vi "Create Array of Tx Message Info.vi"(7 "error in":errorcluster, 8 "1553 channel handles":T7[](array[typedef]) {"terminal status channels" format="%.0x"; "error count channel refs"."wrong sync" format="%.0x"; "error count channel refs"."word" format="%.0x"; "error count channel refs"."unconfigured frames" format="%.0x"; "error count channel refs"."parity" format="%.0x"; "error count channel refs"."monitor" format="%.0x"; "error count channel refs"."Manchester" format="%.0x"; "error count channel refs"."improper number of words" format="%.0x"; "error count channel refs"."general protocol" format="%.0x"; "messages"."Rx status handles" format="%.0x"; "messages"."Tx status handles" format="%.0x"; "messages"."timestamps" format="%.0x"; "messages"."parameters"."RxBC channel handle" format="%.0x"; "messages"."parameters"."RxRT channel handle" format="%.0x"; "messages"."parameters"."Tx channel handle" format="%.0x"}, 9 "hardware handles":T12, 10 "1553 channels":T13[](array[typedef])) -> (0 "error out":errorcluster, 2 "transmitted messages":T1[](array[typedef]), 3 "array of message info":T6[](array[typedef]))   [LabVIEW 2023, in "Ballard MIL-STD-1553 Engine Support.lvlib" / "Custom Device.lvlib"]
uses:
  Custom Device.lvlib
  Shared/1553 Channel.ctl
  Shared/Address.ctl
  Shared/Message Definition.ctl
  Shared/Message Type.ctl
  Shared/Terminal Endpoint.ctl
  Shared/Parameter Definition.ctl
  Hardware Handles.ctl
  Implementation/Execution Unit/1553 Channel Handles.ctl
  Implementation/Execution Unit/Message Handles.ctl
  Implementation/Execution Unit/Parameter Handles.ctl
  <vilib>/NI VeriStand/Custom Device API/Custom Device Item Ref.ctl
  Shared/Error Count Channel Refs.ctl
  Shared/Tx Write Info.ctl
  <vilib>/NI VeriStand/Custom Device API/Custom Device API.lvlib
  Implementation/Execution Unit/Execution Unit.lvclass
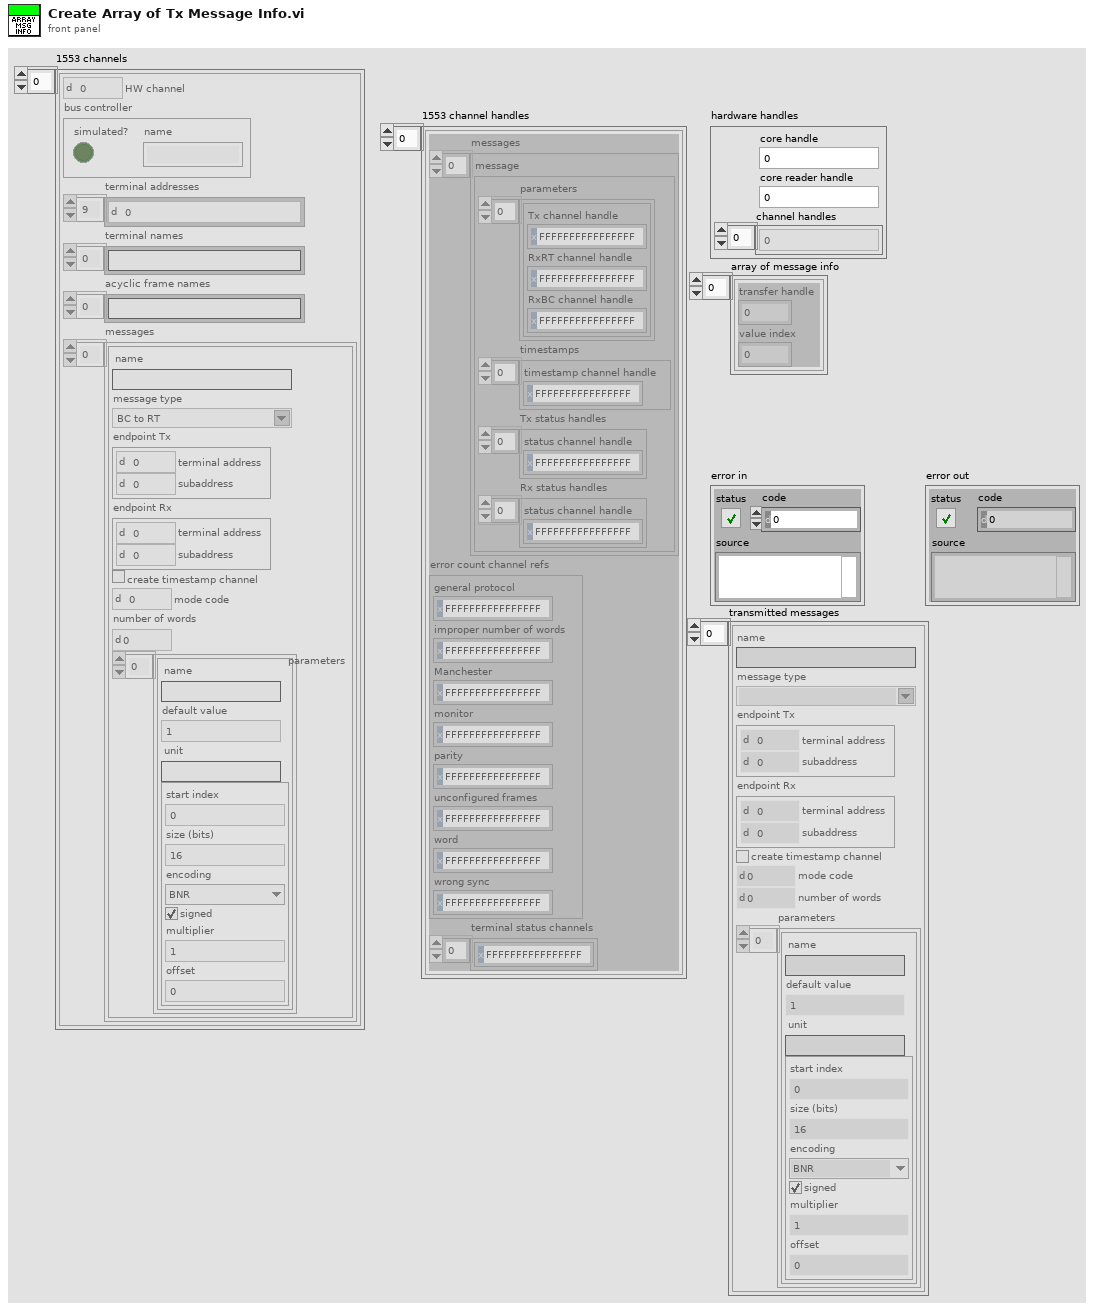
[diagram p1: front panel]
types:
  T1 = typedef "Message Definition.ctl" = cluster{"name":string, "message type":T2, "endpoint Tx":T3, "endpoint Rx":T3, "create timestamp channel":bool, "mode code":u16, "number of words":u16, "parameters":cluster{"name":string, "default value":dbl, "unit":string, "parameter definition":T5}[]}
  T2 = typedef "Message Type.ctl" = string
  T3 = typedef "Terminal Endpoint.ctl" = cluster{"terminal address":T4, "subaddress":T4}
  T4 = typedef "Address.ctl" = u16
  T5 = typedef "Parameter Definition.ctl" = cluster{"start index":i32, "size (bits)":i32, "encoding":enum16{"BNR", "BCD", "Discrete"}, "signed":bool, "multiplier":dbl, "offset":dbl}
  T6 = typedef "Tx Write Info.ctl" = cluster{"transfer handle":u64, "value index":i32}
  T7 = typedef "Ballard MIL-STD-1553 Engine Support.lvlib/Implementation.lvlib/Execution Unit.lvclass/1553 Channel Handles.ctl" = cluster{"messages":T8[], "error count channel refs":T11, "terminal status channels":T10[]}
  T8 = typedef "Ballard MIL-STD-1553 Engine Support.lvlib/Implementation.lvlib/Execution Unit.lvclass/Message Handles.ctl" = cluster{"parameters":T9[], "timestamps":T10[], "Tx status handles":T10[], "Rx status handles":T10[]}
  T9 = typedef "Ballard MIL-STD-1553 Engine Support.lvlib/Implementation.lvlib/Execution Unit.lvclass/Parameter Handles.ctl" = cluster{"Tx channel handle":T10, "RxRT channel handle":T10, "RxBC channel handle":T10}
  T10 = typedef "Custom Device API.lvlib/Custom Device Item Ref.ctl" = u64
  T11 = typedef "Error Count Channel Refs.ctl" = cluster{"general protocol":T10, "improper number of words":T10, "Manchester":T10, "monitor":T10, "parity":T10, "unconfigured frames":T10, "word":T10, "wrong sync":T10}
  T12 = typedef "Ballard MIL-STD-1553 Engine Support.lvlib/Custom Device.lvlib/Hardware Handles.ctl" = cluster{"core handle":u64, "core reader handle":u64, "channel handles":u64[]}
  T13 = typedef "1553 Channel.ctl" = cluster{"HW channel":u16, "bus controller":cluster{"simulated?":bool, "name":string}, "terminal addresses":T4[], "terminal names":string[], "acyclic frame names":string[], "messages":T1[]}
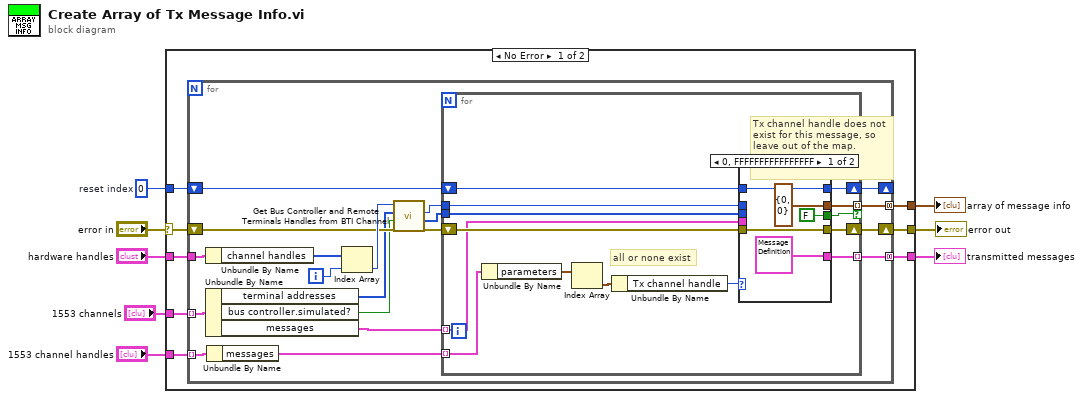
[diagram p0: block diagram]
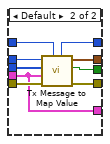
[diagram p2: hidden frame]
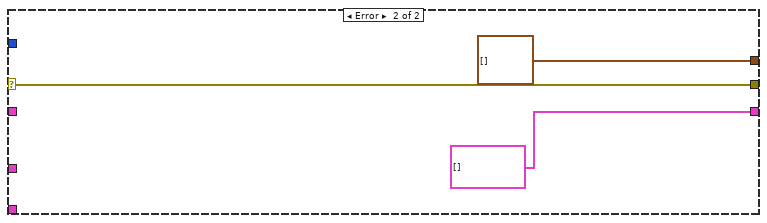
[diagram p3: hidden frame]
diagram:
  w3 = 0  # reset index
  n1 = case shown="No Error" "error in" {
    selector: "error in" -> [w15 w66]
    tunnel: "1553 channels" -> [w12 _]
    tunnel: "hardware handles" -> [w16 _]
    tunnel: [w14 w66] -> w5
    tunnel: "1553 channel handles" -> [w13 _]
    tunnel: w3 -> [w11 _]
    tunnel: [w10 T1[] []] -> w2
    tunnel: [w9 T6[] []] -> w1
    frame No Error {
      n2 = for {
        tunnel: w12 -> [w35] mode=indexing
        tunnel: w16 -> [w33]
        shift-right: [w31] -> w14
        shift-left: w15 -> [w27]
        tunnel: w13 -> [w30] mode=indexing
        shift-right: [w25] -> _
        shift-left: w11 -> [w26]
        tunnel: [w19] -> w10 mode=concatenating
        tunnel: [w18] -> w9 mode=concatenating
        i -> [w20]
        n3 = Unbundle By Name(w33) -> ("channel handles"=w21:u64[])
        n4 = Unbundle By Name(w35) -> ("terminal addresses"=w22:T4[], "bus controller.simulated?"=w17:bool, "messages"=w34:T1[])
        n5 = Unbundle By Name(w30) -> ("messages"=w29:T8[])
        n6 = Index Array(array=w21, index=w20) -> (element=w28:u64)
        n7 = call "Get Bus Controller and Remote Terminals Handles from BTI Channel.vi"("error in"=w27, "bus controller?"=w17, "terminal addresses"=w22, "channel handle in"=w28) -> ("error out"=w32:errorcluster, "remote terminal handles out"=w23:u64[], "bus controller handle out"=w24:u64)  [unwired: 4 in, 1 out]
        n8 = for {
          tunnel: w34 -> [w39] mode=indexing
          shift-right: [w49] -> w31
          shift-left: w32 -> [w42]
          tunnel: w23 -> [w48]
          tunnel: w29 -> [w47] mode=indexing
          tunnel: w24 -> [w43]
          shift-right: [w40] -> w25
          shift-left: w26 -> [w41]
          tunnel: [w37] -> w19 mode=indexing
          tunnel: [w38] -> w18 mode=indexing if=w36
          # "all or none exist"
          n9 = Unbundle By Name(w47) -> ("parameters"=w46:T9[])
          n10 = Index Array(array=w46) -> (element=w45:T9)  [unwired: 1 in]
          n11 = Unbundle By Name(w45) -> ("Tx channel handle"=w44:T10)
          n12 = case shown="0, FFFFFFFFFFFFFFFF" w44 {
            tunnel: w42 -> [w54 w63]
            tunnel: [w54 w62] -> w49
            tunnel: w48 -> [_ w61]
            tunnel: w39 -> [_ w56]
            tunnel: w43 -> [_ w60]
            tunnel: w41 -> [w53 w59]
            tunnel: [w53 w58] -> w40
            tunnel: [T6 {"transfer handle"=0, "value index"=0} ("Tx write info") w57] -> w38
            tunnel: [T1 {"name"="", "message type"="BC to RT", "endpoint Tx"={"terminal address"=0, "subaddress"=0}, "endpoint Rx"={"terminal address"=0, "subaddress"=0}, "create timestamp channel"=FALSE, "mode code"=0, "number of words"=0, "parameters"=[]} w56] -> w37
            tunnel: [FALSE ("valid?") w55] -> w36
            frame 0, -1 {
              # "Tx channel handle does not exist for this message, so leave out of the map."
            }
            frame Default {
              n13 = call "Tx Message to Map Value.vi"("parameter index"=w59, "error in"=w63, "message"=w56, "remote terminal handles"=w61, "bus controller handle"=w60) -> ("error out"=w62:errorcluster, "valid?"=w55:bool, "Tx write info"=w57:T6, "next parameter index"=w58:i32)  [unwired: 3 in]
            }
          }
        }
      }
    }
    frame Error {
    }
  }
  "error out" <- w5
  "array of message info" <- w1
  "transmitted messages" <- w2
